vi "Test PUBREC packet.vi"(8 "error in (no error)":errorcluster) -> (0 "error out":errorcluster)   [LabVIEW 2013]
uses:
  source/Control Packets/PUBREC/PUBREC.lvclass
  source/Control Packets/ControlPacket/ControlPacket.lvclass/ControlPacket.ctl
  source/Control Packets/ControlPacket/ControlPacket.lvclass
  <vilib>/addons/_JKI Toolkits/Caraya/classes/Test/Test.lvclass
  <vilib>/addons/_JKI Toolkits/Caraya/classes/Assert/Assert.lvclass
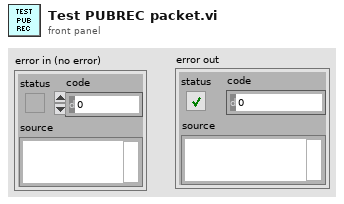
[diagram p1: front panel]
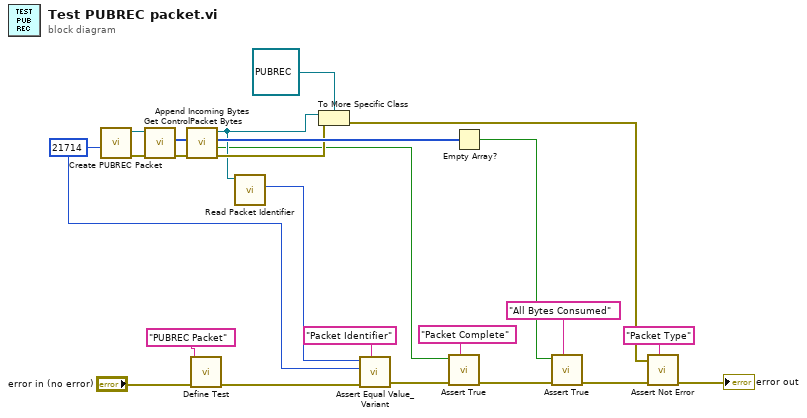
[diagram p0: block diagram]
diagram:
  w5 = u16 21714 ("Packet ID")
  n1 = call "Create PUBREC Packet.vi"("Packet ID"=w5) -> ("error out"=w18:errorcluster, "PUBREC out"=w19:refnum<class "PUBREC.lvclass">)  [unwired: 9 in]
  n2 = call "Get ControlPacket Bytes.vi"("error in (no error)"=w18, "ControlPacket"=w19) -> ("error out"=w22:errorcluster, "Bytes Stream"=w24:u8[])  [unwired: 6 in, 2 out]
  n3 = call "Append Incoming Bytes.vi"("error in (no error)"=w22, "Incoming Packets"=w24) -> ("error out"=w21:errorcluster, "Complete Packet"=w3:bool, "Remaining Packets"=w23:u8[], "ControlPacket"=w20:refnum<class "ControlPacket.lvclass">)  [unwired: 6 in]
  n4 = call <vilib>:"Define Test.vi"("error in (no error)"="error in (no error)", "Label (VI Title)"="PUBREC Packet") -> ("error out"=w11:errorcluster)  [unwired: 9 in]
  n5 = call "Read Packet Identifier.vi"("ControlPacket in"=w20) -> ("Packet Identifier"=w6:u16)  [unwired: 9 in, 1 out]
  n6 = To More Specific Class(target class=refnum<class "PUBREC.lvclass"> refnum ("MQTT_Control_Packets.lvlib:PUBREC.lvclass"), reference=w20, error in=w21) -> (error out=w1:errorcluster)  [unwired: 1 out]
  n7 = call <vilib>:"Assert Equal Value_Variant.vi"("Label"="Packet Identifier" ("Label (VI Title)"), "error in (no error)"=w11, "Y"=w5, "X"=w6) -> ("error out"=w4:errorcluster)  [unwired: 7 in]
  n8 = call <vilib>:"Assert True.vi"("Label"="Packet Complete" ("Label (VI Title)"), "error in (no error)"=w4, "True?"=w3) -> ("error out"=w12:errorcluster)  [unwired: 8 in]
  n9 = Empty Array?(array=w23) -> (empty?=w2:bool)
  n10 = call <vilib>:"Assert True.vi"("Label"="All Bytes Consumed" ("Label (VI Title)"), "error in (no error)"=w12, "True?"=w2) -> ("error out"=w8:errorcluster)  [unwired: 8 in]
  n11 = call <vilib>:"Assert Not Error.vi"("Label"="Packet Type" ("Label (VI Title)"), "error in (no error)"=w8, "Not Error?"=w1) -> ("error out"=→"error out":errorcluster)  [unwired: 8 in]
